vi "7HP_Pre_Analysis_Plugin.vi"() -> ()   [LabVIEW 2021]
uses:
  Globals/Meas_global.vi
  Analysis/7 Hole Probe pressures to UVW/7HP_Global.vi
panel:
  out "UVW chs":i32[](array[numeric])
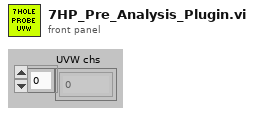
[diagram p1: front panel]
types:
  T1 = typedef "Device ID port info.ctl" = cluster{"Ch No":i16[], "Req Sampling Rate":dbl[], "Port":string, "Index":i32[]}
  T2 = typedef "Analysis_info_cluster.ctl" = cluster{"Colour":u32, "Inst type":T3, "Inst name":string, "Symbol":string, "Code name":string, "Extra Info":string, "Inst Array":T4, "Extra Titles":string[], "Extra Values":string[], "U":dbl, "u^2":dbl, "u^3":dbl, "u^4":dbl, "Skew_u":dbl, "Kurt_u":dbl, "Sd Error in Mean":dbl, "% u'/U":dbl, "X":dbl, "Y":dbl, "Z":dbl, "Timescale integral Estimate":dbl, "Sd Error in Variance":dbl, "Calib File":path, "Calib Constants":dbl[], "Output Position":bool, "Stats":enum16{"None", "Basic", "Full"}, "Av Sampling Rate":dbl, "Av No of Samples":dbl, "Total Meas Time (s)":dbl, "ADAM Ch Name":string, "Max value":dbl, "Min value":dbl, "Req Sample Rate Hz":dbl, "Sync Delay Time (s)":dbl, "Ch No":i16, "Device":string, "Use Latest Calib":bool, "Port":string, "Metadata Ch Names":string[], "Metadata Ch Values":string[], "Label":string}
  T3 = typedef "Inst_type.ctl" = enum16{"Raw voltage", "Raw with zero offsetting", "Propeller anemometer", "Pressure Transducer", "Pitot-static tube", "Hot wire", "Cross wire 1", "Cross wire 2", "Generic Linear", "Generic Polynomial", "Generic BackPoly", "Fast FID", "Thermocouple", "Cold wire", "Pulsed Wire", "LDA Vel", "LDA Tran time", "LDA Arr time", "Microphone"}
  T4 = typedef "Instrument_Array.ctl" = enum16{"PWA", "LDA", "Analogue"}
  T5 = typedef "Time_Trace_Cluster.ctl" = cluster{"Weighting":dbl[], "Voltage":dbl[], "Eng Values":dbl[]}
  T6 = typedef "Cross_Moments_Shift_Cluster.ctl" = cluster{"Stats":dbl[], "Resampled No of Samples":i32, "Resampled delta T":dbl, "Cross Correlation":dbl[]}
  T7 = typedef "Shift_Cluster.ctl" = cluster{"Stats":dbl[], "Spectra_Auto":dbl[], "Histogram":dbl[], "Hist Max":dbl, "Hist Min":dbl, "No of Samples":i32, "No in plume":i32, "Weight sum":dbl, "No Of Hist bins":i32, "TimeTrace Max":dbl, "Time Trace Min":dbl, "Trace St Deviation":dbl}
  T8 = typedef "Correlation_cluster1.ctl" = cluster{"U inst":string, "uw":dbl, "u^2w":dbl, "uw^2":dbl, "uw/u'w'":dbl, "W inst":string, "uw^3":dbl, "u^3w":dbl, "u^2w^2":dbl, "Index U":i32, "Index W":i32, "Error info":string[], "Paired Sampling Rate (Hz)":dbl, "u^2 Paired":dbl, "w^2 Paired":dbl, "Time Window (ms)":dbl}
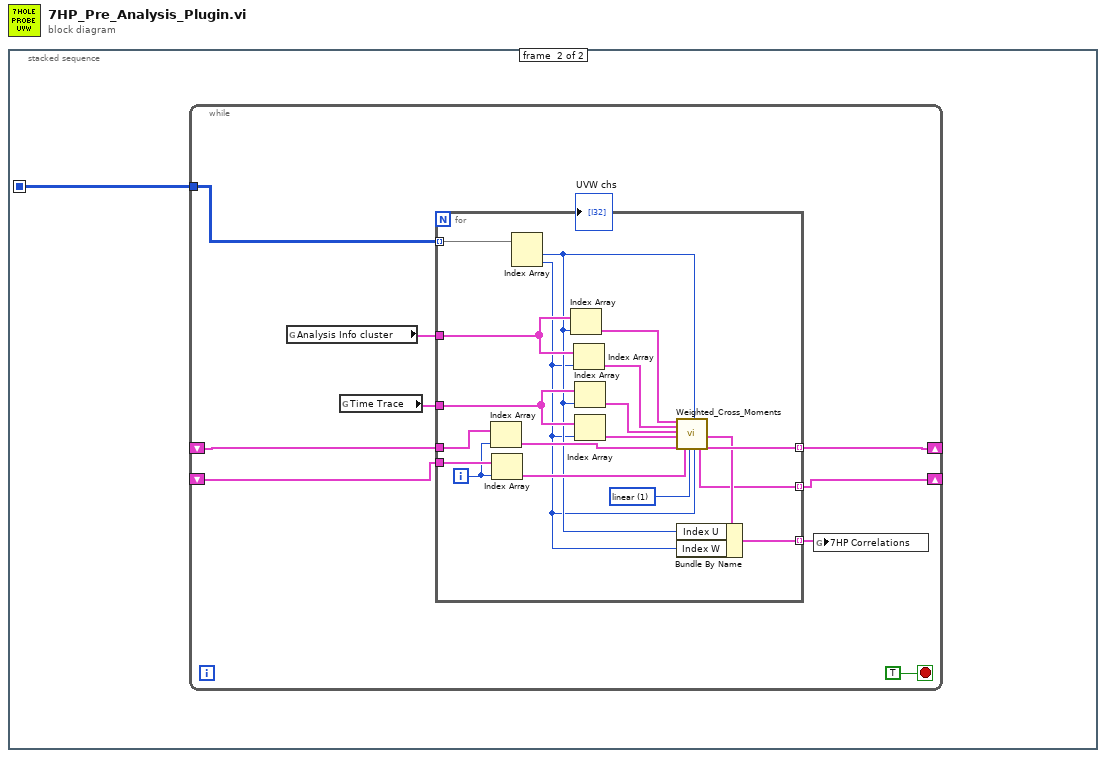
[diagram p0: block diagram]
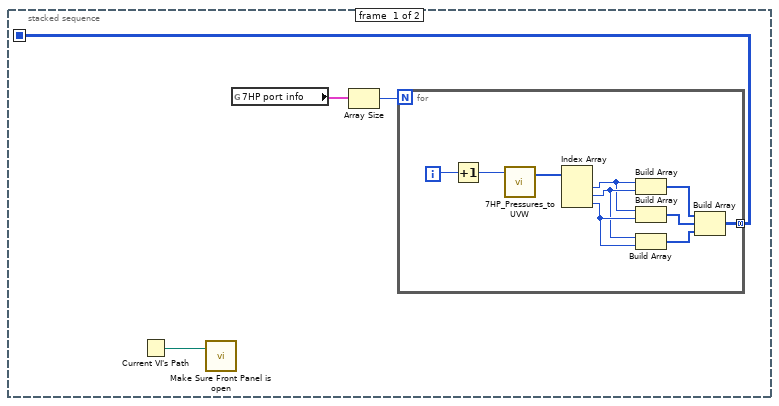
[diagram p2: hidden frame]
diagram:
  n1 = stacked-sequence {
    seq-local: [w3 _] -> [_ w15]
    frame #0 {
      n2 = Current VI's Path() -> (path=w1:path)
      n3 = call "Make Sure Front Panel is open.vi"("path"=w1) -> ()
      n4 = global read "7HP_Global.vi" "7HP port info"() -> (w2:T1[])
      n5 = Array Size(array=w2) -> (size(s)=w4:i32)
      n6 = for {
        N: w4 -> [_]
        tunnel: [w5] -> w3 mode=concatenating
        i -> [w14]
        n7 = Increment(x=w14) -> (x+1=w13:i32)
        n8 = call "7HP_Pressures_to UVW.vi"("Probe Number"=w13) -> ("UVW chs"=w6:i32[])  [unwired: 2 in]
        n9 = Index Array(array=w6) -> (element #1=w7:i32, element #2=w8:i32, element #3=w9:i32)  [unwired: 3 in]
        n10 = Build Array(w7, w8) -> (w10:i32[])
        n11 = Build Array(w7, w9) -> (w11:i32[])
        n12 = Build Array(w8, w9) -> (w12:i32[])
        n13 = Build Array(w10, w11, w12) -> (w5:i32[][])
      }
    }
    frame #1 {
      n14 = while {
        shift-right: [w23] -> _
        shift-left: _ -> [w21]
        shift-right: [w22] -> _
        shift-left: _ -> [w20]
        tunnel: w15 -> [w19]
        stop <- TRUE stop-if-true
        n15 = global read "Meas_global.vi" "Analysis Info cluster"() -> (w18:T2[])
        n16 = global read "Meas_global.vi" "Time Trace"() -> (w24:T5[])
        n17 = for {
          tunnel: w19 -> [w43] mode=indexing
          tunnel: w18 -> [w41]
          tunnel: [w39] -> w23 mode=indexing
          tunnel: w21 -> [w38]
          tunnel: [w35] -> w16 mode=indexing
          tunnel: w24 -> [w34]
          tunnel: [w29] -> w22 mode=indexing
          tunnel: w20 -> [w28]
          i -> [w27]
          w31 = 1 items=["nearest", "linear", "spline", "cubic Hermite", "Lagrange"] ("interp. method")
          n18 = Index Array(array=w38, index=w27) -> (element=w37:T6)
          n19 = Index Array(array=w28, index=w27) -> (element=w30:T7)
          n20 = Index Array(array=w43) -> (element #1=w26:i32, element #2=w25:i32)  [unwired: 2 in]
          n21 = Index Array(array=w41, index=w26) -> (element=w42:T2)
          n22 = Index Array(array=w41, index=w25) -> (element=w40:T2)
          n23 = Index Array(array=w34, index=w26) -> (element=w33:T5)
          n24 = Index Array(array=w34, index=w25) -> (element=w32:T5)
          n25 = call "Weighted_Cross_Moments.vi"("AI Cluster 1"=w42, "AI Cluster 2"=w40, "Time Cluster 1"=w33, "Time Cluster 2"=w32, "Shift Cluster In"=w37, "Shift Input"=w30, "interp. method"=w31, "Index1"=w26, "Index2"=w25) -> ("Shift Output"=w29:T7, "output cluster"=w36:T8, "Shift Cluster Out"=w39:T6)  [unwired: 8 in]
          n26 = Bundle By Name(cluster=w36, "Index U"=w26, "Index W"=w25) -> (w35:T8)
        }
        n27 = global write "7HP_Global.vi" "7HP Correlations"(w16) -> ()
      }
    }
  }
